vi "get_power_reading.vi"(0 "Power Meter Connection Data In":T3, 2 "Q Laser Data?":bool, 11 "Laser Power Q In":T1) -> (4 "Power Meter Connection Data Out":T3, 12 "error out":errorcluster, 14 "Data Out":T2, 15 "Laser Power Q Out":T1)   [LabVIEW 2023]
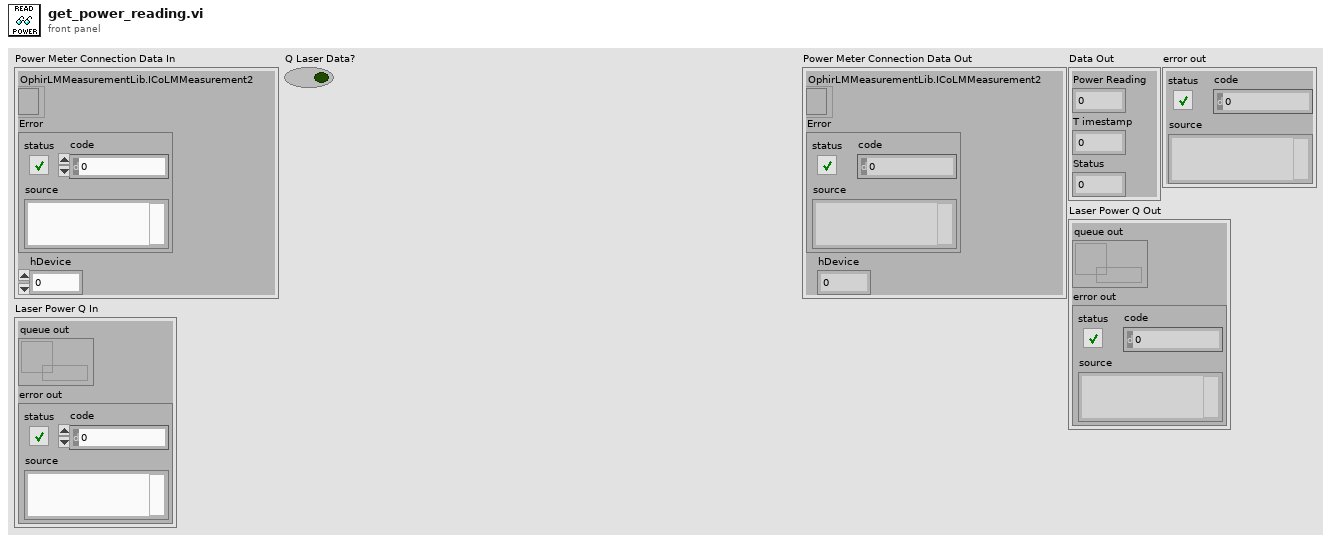
[diagram p1: front panel]
types:
  T1 = cluster{"queue out":refnum<queue>, "error out":errorcluster}
  T2 = cluster{"Power Reading ":dbl, "T imestamp":dbl, "Status":i32}
  T3 = cluster{"OphirLMMeasurementLib.ICoLMMeasurement2":refnum<k7>, "Error":errorcluster, "hDevice":i32}
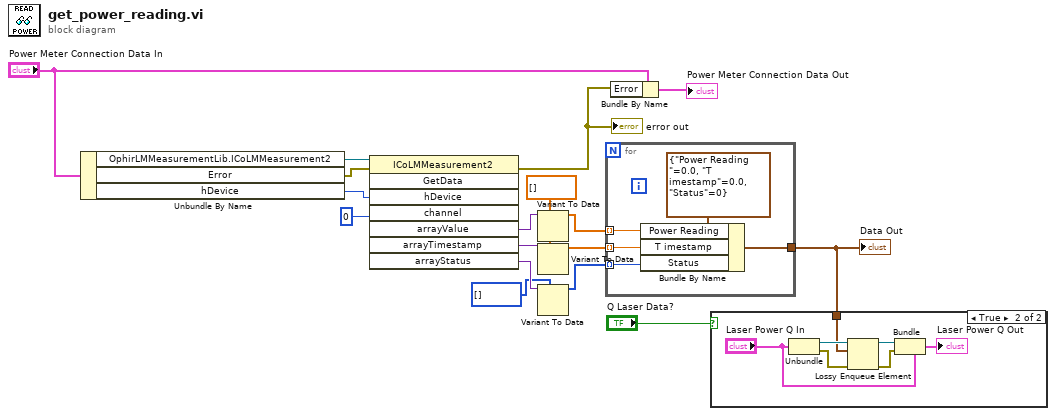
[diagram p0: block diagram]
diagram:
  w16 = dbl[] []
  n1 = Unbundle By Name("Power Meter Connection Data In") -> ("OphirLMMeasurementLib.ICoLMMeasurement2"=w8:refnum<k7>, "Error"=w7:errorcluster, "hDevice"=w6:i32)
  n2 = invoke class="ICoLMMeasurement2" method="GetData"(reference=w8, error in=w7, "hDevice"=w6, "channel"=0) -> (error out=w1:errorcluster, "arrayValue"=w15:variant, "arrayTimestamp"=w14:variant, "arrayStatus"=w13:variant)  [unwired: 4 in, 4 out]
  "error out" <- w1
  n3 = Variant To Data(type=w16, Variant=w15) -> (data=w12:dbl[])  [unwired: 1 in, 1 out]
  n4 = Variant To Data(type=w16, Variant=w14) -> (data=w11:dbl[])  [unwired: 1 in, 1 out]
  n5 = Variant To Data(type=i32[] [], Variant=w13) -> (data=w10:i32[])  [unwired: 1 in, 1 out]
  n6 = for {
    tunnel: w12 -> [w21] mode=indexing
    tunnel: w11 -> [w20] mode=indexing
    tunnel: w10 -> [w19] mode=indexing
    tunnel: [w18] -> w4
    n7 = Bundle By Name(cluster=T2 {"Power Reading "=0.0, "T imestamp"=0.0, "Status"=0}, "Power Reading"=w21, "T imestamp"=w20, "Status"=w19) -> (w18:T2)
  }
  "Data Out" <- w4
  n8 = Bundle By Name(cluster="Power Meter Connection Data In", "Error"=w1) -> (→"Power Meter Connection Data Out":T3)
  n9 = case shown="True" "Q Laser Data?" {
    tunnel: w4 -> [_ w27]
    frame False {
    }
    frame True {
      n10 = Unbundle("Laser Power Q In") -> ("queue out"=w29:refnum<queue>, "error out"=w28:errorcluster)
      n11 = Lossy Enqueue Element(queue=w29, element=w27, error in (no error)=w28) -> (queue out=w26:refnum<queue>, error out=w25:errorcluster)  [unwired: 2 out]
      n12 = Bundle(cluster="Laser Power Q In", "queue out"=w26, "error out"=w25) -> (→"Laser Power Q Out":T1)
    }
  }
